vi "startup.vi"() -> (0 "System parameters":T1, 1 "Active process at IC6":i32, 2 "Stop?":bool, 3 "Elements+Rates ring items":cluster{"Element":string, "Value":u16}[](array[cluster]))   [LabVIEW 2012]
uses:
  <vilib>/Utility/file.llb/Read From Spreadsheet File (string).vi
  elements.gbl
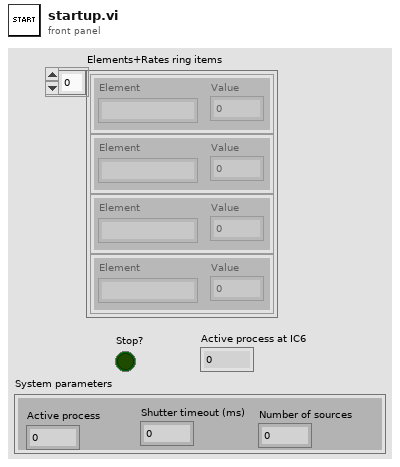
[diagram p1: front panel]
types:
  T1 = cluster{"Active process":i32, "Shutter timeout (ms)":u32, "Number of sources":i32}
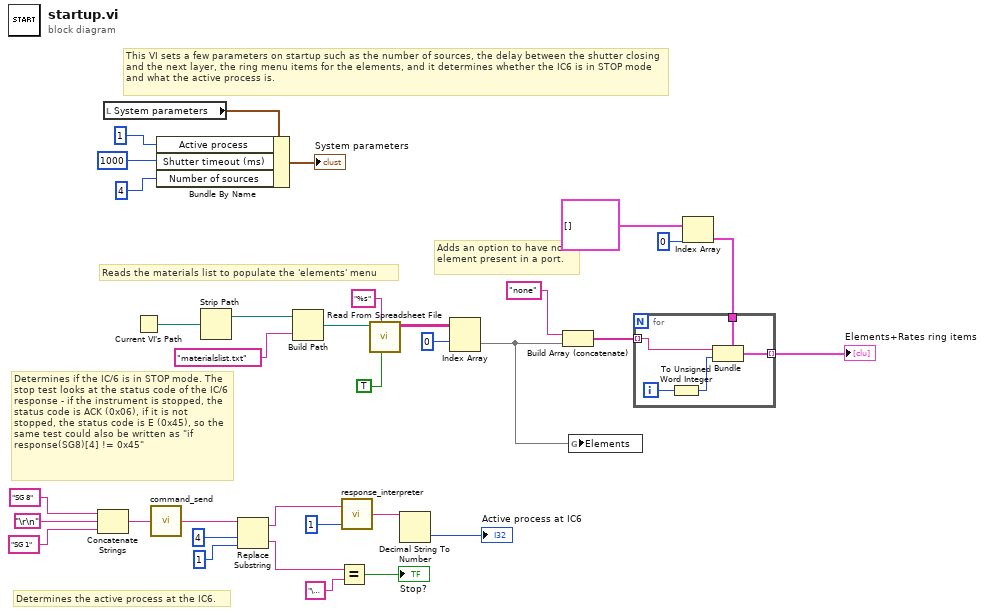
[diagram p0: block diagram]
diagram:
  # "This VI sets a few parameters on startup such as the number of sources, the delay between the shutter closing and the next layer, the ring menu items for the elements, and it determines whether the IC6 is in STOP mode and what the active process is."
  # "Determines the active process at the IC6."
  # "Determines if the IC/6 is in STOP mode. The stop test looks at the status code of the IC/6 response - if the instrument is stopped, the status code is ACK (0x06), if it is not stopped, the status code is E (0x45), so the same test could also be written as \"if response(SG8)[4] != 0x45\""
  # "Reads the materials list to populate the 'elements' menu"
  # "Adds an option to have no element present in a port."
  n1 = Concatenate Strings("SG 8", "\r\n", "SG 1") -> (w16:string)
  n2 = local read "System parameters"() -> (w4:T1)
  n3 = Current VI's Path() -> (path=w34:path)
  n4 = call "command_send.vi"("Commands"=w16) -> ("Response"=w19:string)
  n5 = Bundle By Name(cluster=w4, "Active process"=1, "Shutter timeout (ms)"=u32 1000, "Number of sources"=u32 4) -> (→"System parameters":T1)
  n6 = Strip Path(path=w34) -> (stripped path=w33:path)  [unwired: 1 out]
  n7 = Replace Substring(2:1, 3:4, 5:w19) -> (0:w5:string, 1:w6:string)  [unwired: 1 in]
  n8 = Build Path(base path=w33, name or relative path="materialslist.txt") -> (appended path=w31:path)
  n9 = Equal?(x=w5, y="\u0006") -> (x = y?=→"Stop?":bool)
  n10 = call "response_interpreter.vi"("Response type"=u16 1, "Response hex"=w6) -> ("Response (readable)"=w9:string)
  n11 = call-poly <vilib>:"Read From Spreadsheet File.vi"("transpose (no:F)"=TRUE, "format (%s)"="%s", "file path (dialog if empty)"=w31) -> ("all rows"=w28:string[][])  [unwired: 4 in, 4 out]
  n12 = Decimal String To Number(string=w9) -> (number=→"Active process at IC6":i32)  [unwired: 2 in, 1 out]
  n13 = Index Array(array=w28, index (row)=0) -> (element=w21:string[])  [unwired: 1 in]
  n14 = Build Array (concatenate)("none", w21) -> (w22:string[])
  n15 = global write "elements.gbl" "Elements"(w21) -> ()
  n16 = Index Array(array=cluster{"String":string, "Value":u16}[] [] ("Strings And Values []"), index=0) -> (element=w23:cluster{"String":string, "Value":u16})
  n17 = for {
    tunnel: w22 -> [w38] mode=indexing
    tunnel: [w36] -> w26 mode=indexing
    tunnel: w23 -> [w35]
    i -> [w39]
    n18 = To Unsigned Word Integer(number=w39) -> (unsigned 16bit integer=w37:u16)
    n19 = Bundle(cluster=w35, "String"=w38, "Value"=w37) -> (w36:cluster{"String":string, "Value":u16})
  }
  "Elements+Rates ring items" <- w26
